vi "UWGN ident.vi"() -> ()   [LabVIEW 2015]
uses:
  <vilib>/Platform/TimedLoop/XDataNode/timing_clust.ctl
  <vilib>/Platform/TimedLoop/XDataNode/nitl_modes.ctl
  <vilib>/Platform/TimedLoop/XDataNode/wakeup.ctl
  <vilib>/FPGAPlugInAG/myRIO-1900/niLvFpga_Open_myRIO-1900.vi
  <vilib>/rvi/interface/common/dynamic/niFpgaDynamicAddResources.vi
  <vilib>/Utility/file.llb/Write Delimited Spreadsheet (DBL).vi
  <vilib>/Utility/error.llb/Error Cluster From Error Code.vi
  <vilib>/rvi/errors/niLvFpgaAdjustHostInterfaceError.vi
  <vilib>/FPGAPlugInAG/Dynamic/niLvFpga_Close_Dynamic.vi
  <vilib>/rvi/interface/nirviOpenFPGA/nirviOpenFPGA.xnode
  FPGA Bitfiles/ViconProj_FPGATarget_CurrentControlle_KJVtLDFLiQk.lvbitx
  Misc/Current Controller.vi
  <vilib>/Platform/TimedLoop/XDataNode/XDataNode.xnode
  <vilib>/rvi/interface/nirviReadWriteControl/nirviReadWriteControl.xnode
  <vilib>/rvi/interface/nirviCloseFPGA/nirviCloseFPGA.xnode
  <vilib>/rvi/interface/Simulation/niFpgaSimulationCallBeginRW.vi
  <vilib>/Analysis/NI_AALBase.lvlib
  <vilib>/Platform/TimedLoop/XDataNode/XDNodeRunTimeDep.lvlib
  NiFpgaLv.dll
panel:
  in  "Stop":bool
  in  "Tab Control":enum32{"Monitor"}(tab)
  out "GU Wave":dbl[](graph)
  out "Sensor":dbl(graph)
  out "FPGA Status":bool
  out "FPGA TImed Loop error":errorcluster
  out "FPGA Loop error":errorcluster
  out "UWGN Error":errorcluster
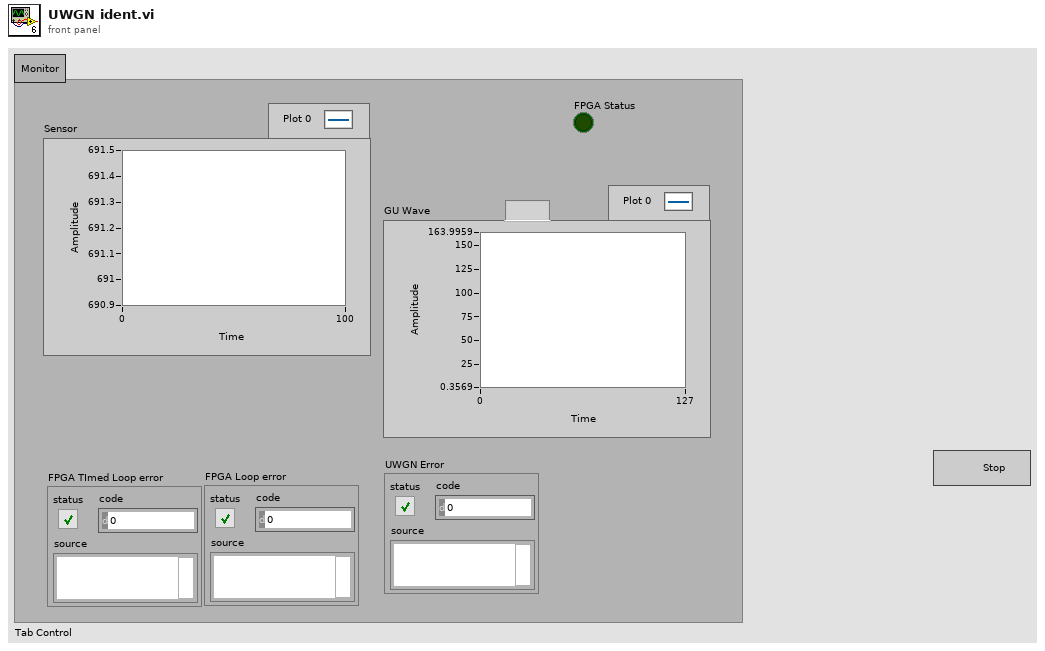
[diagram p1: front panel]
types:
  T1 = typedef "XDNodeRunTimeDep.lvlib/timing_clust.ctl" = cluster{"Expected End [f-1]":u64, "Actual End [f-1]":u64, "Finished Late? [f-1]":bool, "Expected End [i-1]":u64, "Actual End [i-1]":u64, "Finished Late? [i-1]":bool, "Expected Start [i]":u64, "Actual Start [i]":u64, "Expected Start [f]":u64, "Actual Start [f]":u64, "Source Name":string, "Structure Name":string, "Period":i64, "Deadline":i64, "Offset":i64, "Start":i64, "Priority":i32, "Timeout":i32, "Mode":T2, "Wakeup Reason":T3, "Error":errorcluster, "Source Type":string, "Secondary Source Type":string, "Global End Time":u64, "Global Start Time":u64, "Frame Duration":u64, "Iteration Duration":u64, "Assigned CPU":i32, "I/O Scan Engine Mode":u32}
  T2 = typedef "XDNodeRunTimeDep.lvlib/nitl_modes.ctl" = enum32{"No Change", "Process missed periods, maintain original phase", "Discard missed periods, maintain original phase", "Process missed periods, ignore original phase", "Discard missed periods, ignore original phase"}
  T3 = typedef "XDNodeRunTimeDep.lvlib/wakeup.ctl" = enum32{"Normal", "Aborted", "Asynchronous wakeup", "Timing source error", "Timed loop error", "Timeout"}
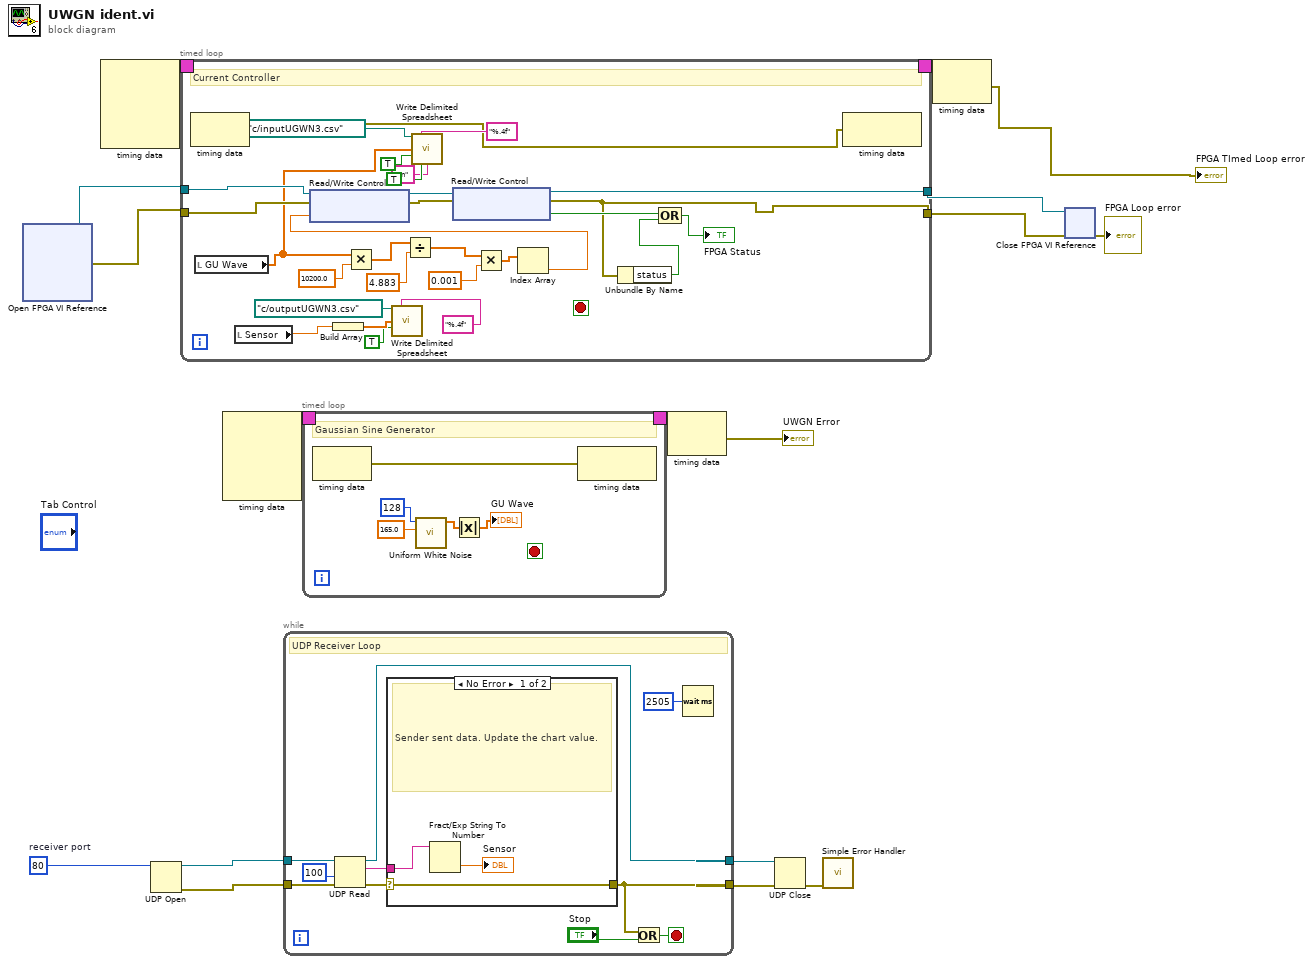
[diagram p0: block diagram]
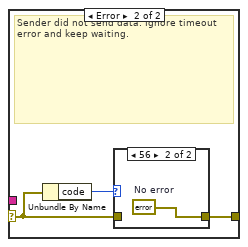
[diagram p2: hidden frame]
diagram:
  w8 = u16 80  # receiver port
  n1 = xnode "Open FPGA VI Reference"() -> ("FPGA VI Reference Out"=w17:refnum<k20>, "error out"=w16:errorcluster)  [unwired: 2 in]
  n2 = node-c288() -> (w5:T1)  [unwired: 4 in]
  n3 = UDP Open(11:w8) -> (port=w9:refnum<k16>, 0:w10:errorcluster)  [unwired: 4 in, 1 out]
  n4 = timed-loop {
    tunnel: w17 -> [w45]
    tunnel: w16 -> [w44]
    tunnel: [w36] -> w15
    tunnel: [w33] -> w14
    timing: w5 -> [_]
    timing-out: [_] -> w4
    stop <- _ stop-if-true
    # "Current Controller"
    n5 = node-c288() -> (w21:errorcluster)  [unwired: 1 in]
    n6 = local read "GU Wave"() -> (w18:dbl[])
    n7 = local read "Sensor"() -> (w27:dbl)
    n8 = Build Array(w27) -> (w28:dbl[])
    n9 = Multiply(x=w18, y=10200.0) -> (x*y=w40:dbl[])
    n10 = call-poly <vilib>:"Write Delimited Spreadsheet.vi"("file path (dialog if empty)"=path "c:/outputUGWN3.csv", "format (%.3f)"="%.4f", "1D data"=w28, "append to file? (F)"=TRUE) -> ()  [unwired: 10 in, 2 out]
    n11 = Divide(x=w40, y=4.883) -> (x/y=w42:dbl[])
    n12 = call-poly <vilib>:"Write Delimited Spreadsheet.vi"("file path (dialog if empty)"=path "c:/inputUGWN3.csv", "format (%.3f)"="%.4f" ("format (%d)"), "1D data"=w18, "append to file? (F)"=TRUE, "transpose? (F)"=TRUE, "delimiter (\\t)"="\\n" ("delimiter (\\t)")) -> ()  [unwired: 8 in, 2 out]
    n13 = Multiply(x=w42, y=0.001) -> (x*y=w23:dbl[])
    n14 = Index Array(array=w23) -> (element=w22:dbl)  [unwired: 1 in]
    n15 = xnode "Read/Write Control"("FPGA VI Reference In"=w45, "error in"=w44, "DAC Inlet Valve"=w22) -> ("FPGA VI Reference Out"=w38:refnum<k20>, "error out"=w37:errorcluster)
    n16 = xnode "Read/Write Control"("FPGA VI Reference In"=w38, "error in"=w37) -> ("FPGA VI Reference Out"=w36:refnum<k20>, "error out"=w33:errorcluster, "Inlet Overflow?"=w34:bool)
    n17 = Unbundle By Name(w33) -> ("status"=w35:bool)
    n18 = Compound Arithmetic op=OR(w34, w35) -> (→"FPGA Status":bool)
    n19 = node-c288(w21) -> ()  [unwired: 1 out]
  }
  n20 = node-c288() -> (w7:T1)  [unwired: 4 in]
  n21 = while {
    tunnel: w9 -> [w60]
    tunnel: [w52] -> w13
    tunnel: w10 -> [w57]
    tunnel: [w53] -> w11
    stop <- w58 stop-if-true
    # "UDP Receiver Loop"
    n22 = UDP Read(connection ID=w60, timeout ms (25000)=100, 8:w57) -> (data out=w55:string, error out=w54:errorcluster, 3:w52:refnum<k16>)  [unwired: 3 out]
    n23 = case shown="No Error" w54 {
      selector: w54 -> [w61 w65]
      tunnel: w55 -> [w63 _]
      tunnel: [w61 w64] -> w53
      frame No Error {
        # "Sender sent data. Update the chart value."
        n24 = Fract/Exp String To Number(string=w63) -> (number=→"Sensor":dbl)  [unwired: 3 in, 1 out]
      }
      frame Error {
        # "Sender did not send data. Ignore timeout error and keep waiting."
        n25 = Unbundle By Name(w65) -> ("code"=w66:i32)
        n26 = case shown="56" w66 {
          tunnel: w65 -> [w67 _]
          tunnel: [w67 w68] -> w64
          frame Default {
          }
          frame 56 {
            w68 = errorcluster {"status"=FALSE, "code"=0, "source"=""}  # No error
          }
        }
      }
    }
    n27 = Or(x=w53, y="Stop") -> (x .or. y?=w58:bool)
    n28 = Wait (ms)(milliseconds to wait=u32 2505) -> ()  [unwired: 1 out]
  }
  n29 = timed-loop {
    timing: w7 -> [_]
    timing-out: [_] -> w6
    stop <- _ stop-if-true
    # "Gaussian Sine Generator"
    n30 = node-c288() -> (w69:errorcluster)  [unwired: 1 in]
    n31 = call <vilib>:"Uniform White Noise.vi"("amplitude"=165.0, "samples"=128) -> ("uniform white noise"=w71:dbl[])  [unwired: 8 in, 1 out]
    n32 = Absolute Value(x=w71) -> (abs(x)=→"GU Wave":dbl[])
    n33 = node-c288(w69) -> ()  [unwired: 1 out]
  }
  n34 = node-c288(w6) -> (→"UWGN Error":errorcluster)
  n35 = UDP Close(connection ID=w13, 8:w11) -> (error out=w12:errorcluster)  [unwired: 1 out]
  n36 = call <vilib>:"Simple Error Handler.vi"("error in (no error)"=w12) -> ()  [unwired: 1 in, 8 out]
  n37 = node-c288(w4) -> (→"FPGA TImed Loop error":errorcluster)
  n38 = xnode "Close FPGA VI Reference"("FPGA VI Reference In"=w15, "error in"=w14) -> ("error out"=→"FPGA Loop error":errorcluster)
